vi "Write time test.vi"(7 "Map id":i32, 8 "Error In":errorcluster, 10 "Data":dbl[](array[numeric]), 11 "Indices":i32[](array[numeric])) -> (0 "Error Out":errorcluster, 3 "dt":dbl)   [LabVIEW 2018]
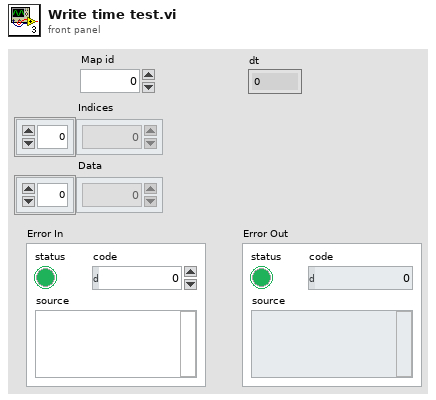
[diagram p1: front panel]
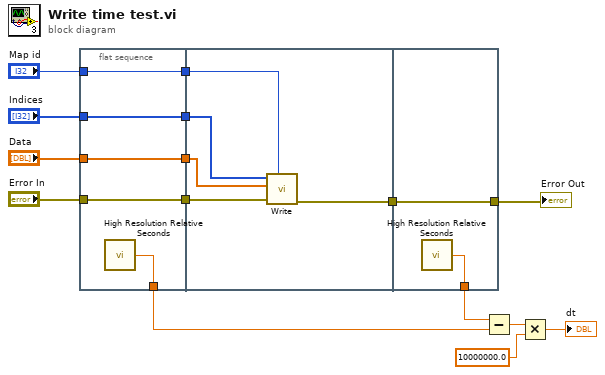
[diagram p0: block diagram]
diagram:
  n1 = flat-sequence {
    tunnel: [w20] -> w4
    tunnel: [w19] -> w15
    tunnel: "Error In" -> [w19]
    tunnel: [w18] -> w11
    tunnel: "Data" -> [w18]
    tunnel: "Indices" -> [w17]
    tunnel: [w17] -> w8
    tunnel: "Map id" -> [w16]
    tunnel: [w16] -> w6
    tunnel: w15 -> [w25]
    tunnel: [w24] -> w13
    tunnel: w11 -> [w23]
    tunnel: w8 -> [w22]
    tunnel: w6 -> [w21]
    tunnel: [w27] -> w5
    tunnel: w13 -> [w26]
    tunnel: [w26] -> w12
    frame #0 {
      n2 = call <vilib>:"High Resolution Relative Seconds.vi"() -> ("relative seconds"=w20:dbl)
    }
    frame #1 {
      n3 = call "Write.vi"("Map id"=w21, "Error In"=w25, "Data"=w23, "Indices"=w22) -> ("Error Out"=w24:errorcluster)  [unwired: 7 in]
    }
    frame #2 {
      n4 = call <vilib>:"High Resolution Relative Seconds.vi"() -> ("relative seconds"=w27:dbl)
    }
  }
  n5 = Subtract(x=w5, y=w4) -> (x-y=w3:dbl)
  n6 = Multiply(x=w3, y=10000000.0) -> (x*y=→"dt":dbl)
  "Error Out" <- w12
